vi "NI 5772 (AC) - Digitizer_(FPGA)AveragingTesting.vi"() -> ()   [LabVIEW 2020]
doc: "Example Description:\nThis example demonstrates how to enable Time Interleaved Sampling with the NI 5772 adapter module to achieve a sampling rate of 1.6GS/s. This example continuously acquires records of analog input data from the NI 5772 adapter module. It allows you to select an AI channel, trigger type, and record size. This VI must be compiled before it is run. \n\nRunning the VI:\nThis VI must be run from the NI 5772 - Getting Started (Host).vi. Refer to the host VI documentation for steps regarding running and configuring the FPGA VI. \n\nExecution Steps:\nRefer to the Block Diagram of this VI for execution comments."
uses:
  Controls/AI Trigger Type.ctl
  Controls/Aquire State.ctl
panel:
  in  "Trigger":bool=TRUE
  out "Trigger Count":u32
  out "Read Size (Host)":u16=512 caption="Samples Per Trigger" min=1 step=1
  in  "TrigIn Simulate":bool
  in  "vi/nGenTrig":bool
  in  "Arm Trigger":bool
  out "F to H FIFO Overflow?":bool caption="FIFO Overflow?"
  out "DataAlignmentFIFO":bool
  out "Aq to Trans FIFO Overflow?":bool caption="FIFO Overflow?"
  in  "Requested Samples Per Pixel":u16=512 caption="Samples Per Trigger" min=1 step=1
  in  "AvgCount_powerOf2":i16=1
  in  "Delay (us)":sgl
  in  "WaveSampleCount":sgl=256.0 format="%#_13g"
  in  "Wave Sampling Rate":sgl=200000000.0 format="%#_6p"
  in  "Trigger Level":i16
  in  "Trigger Type":T1
  out "AvgCount":u16=1
  out "Delay after Trig [cycles]":u16
  out "1/8th Samples Per Trigger":u16=512 caption="Samples Per Trigger" min=1 step=1
  out "WaitForWave\nCompletion [cycles]":u16
  in  "User Command Commit":bool
  in  "User Command":u8
  out "User Command Idle":bool
  out "User Command Status":u8
  in  "User Data 0":u16
  in  "User Data 1":u8
  out "PLL Locked":bool
  out "User Error":bool
  out "Configured?":bool
  # "Trigger Settings"
  # "FIFO Status"
  # "Analog Input"
  # "Clock Configuration"
  # "Resource Configuration"
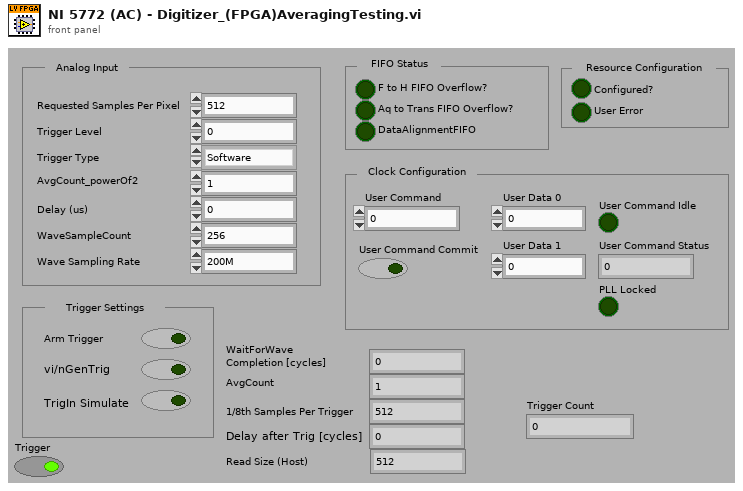
[diagram p1: front panel]
types:
  T1 = typedef "AI Trigger Type.ctl" = enum8{"Software", "Data Edge"}
  T2 = typedef "Aquire State.ctl" = enum8{"Idle", "Wait for Trigger", "AlignWave", "Hold Aquire", "Acquire", "WaitForWaveCompletion", "CheckAvg"}
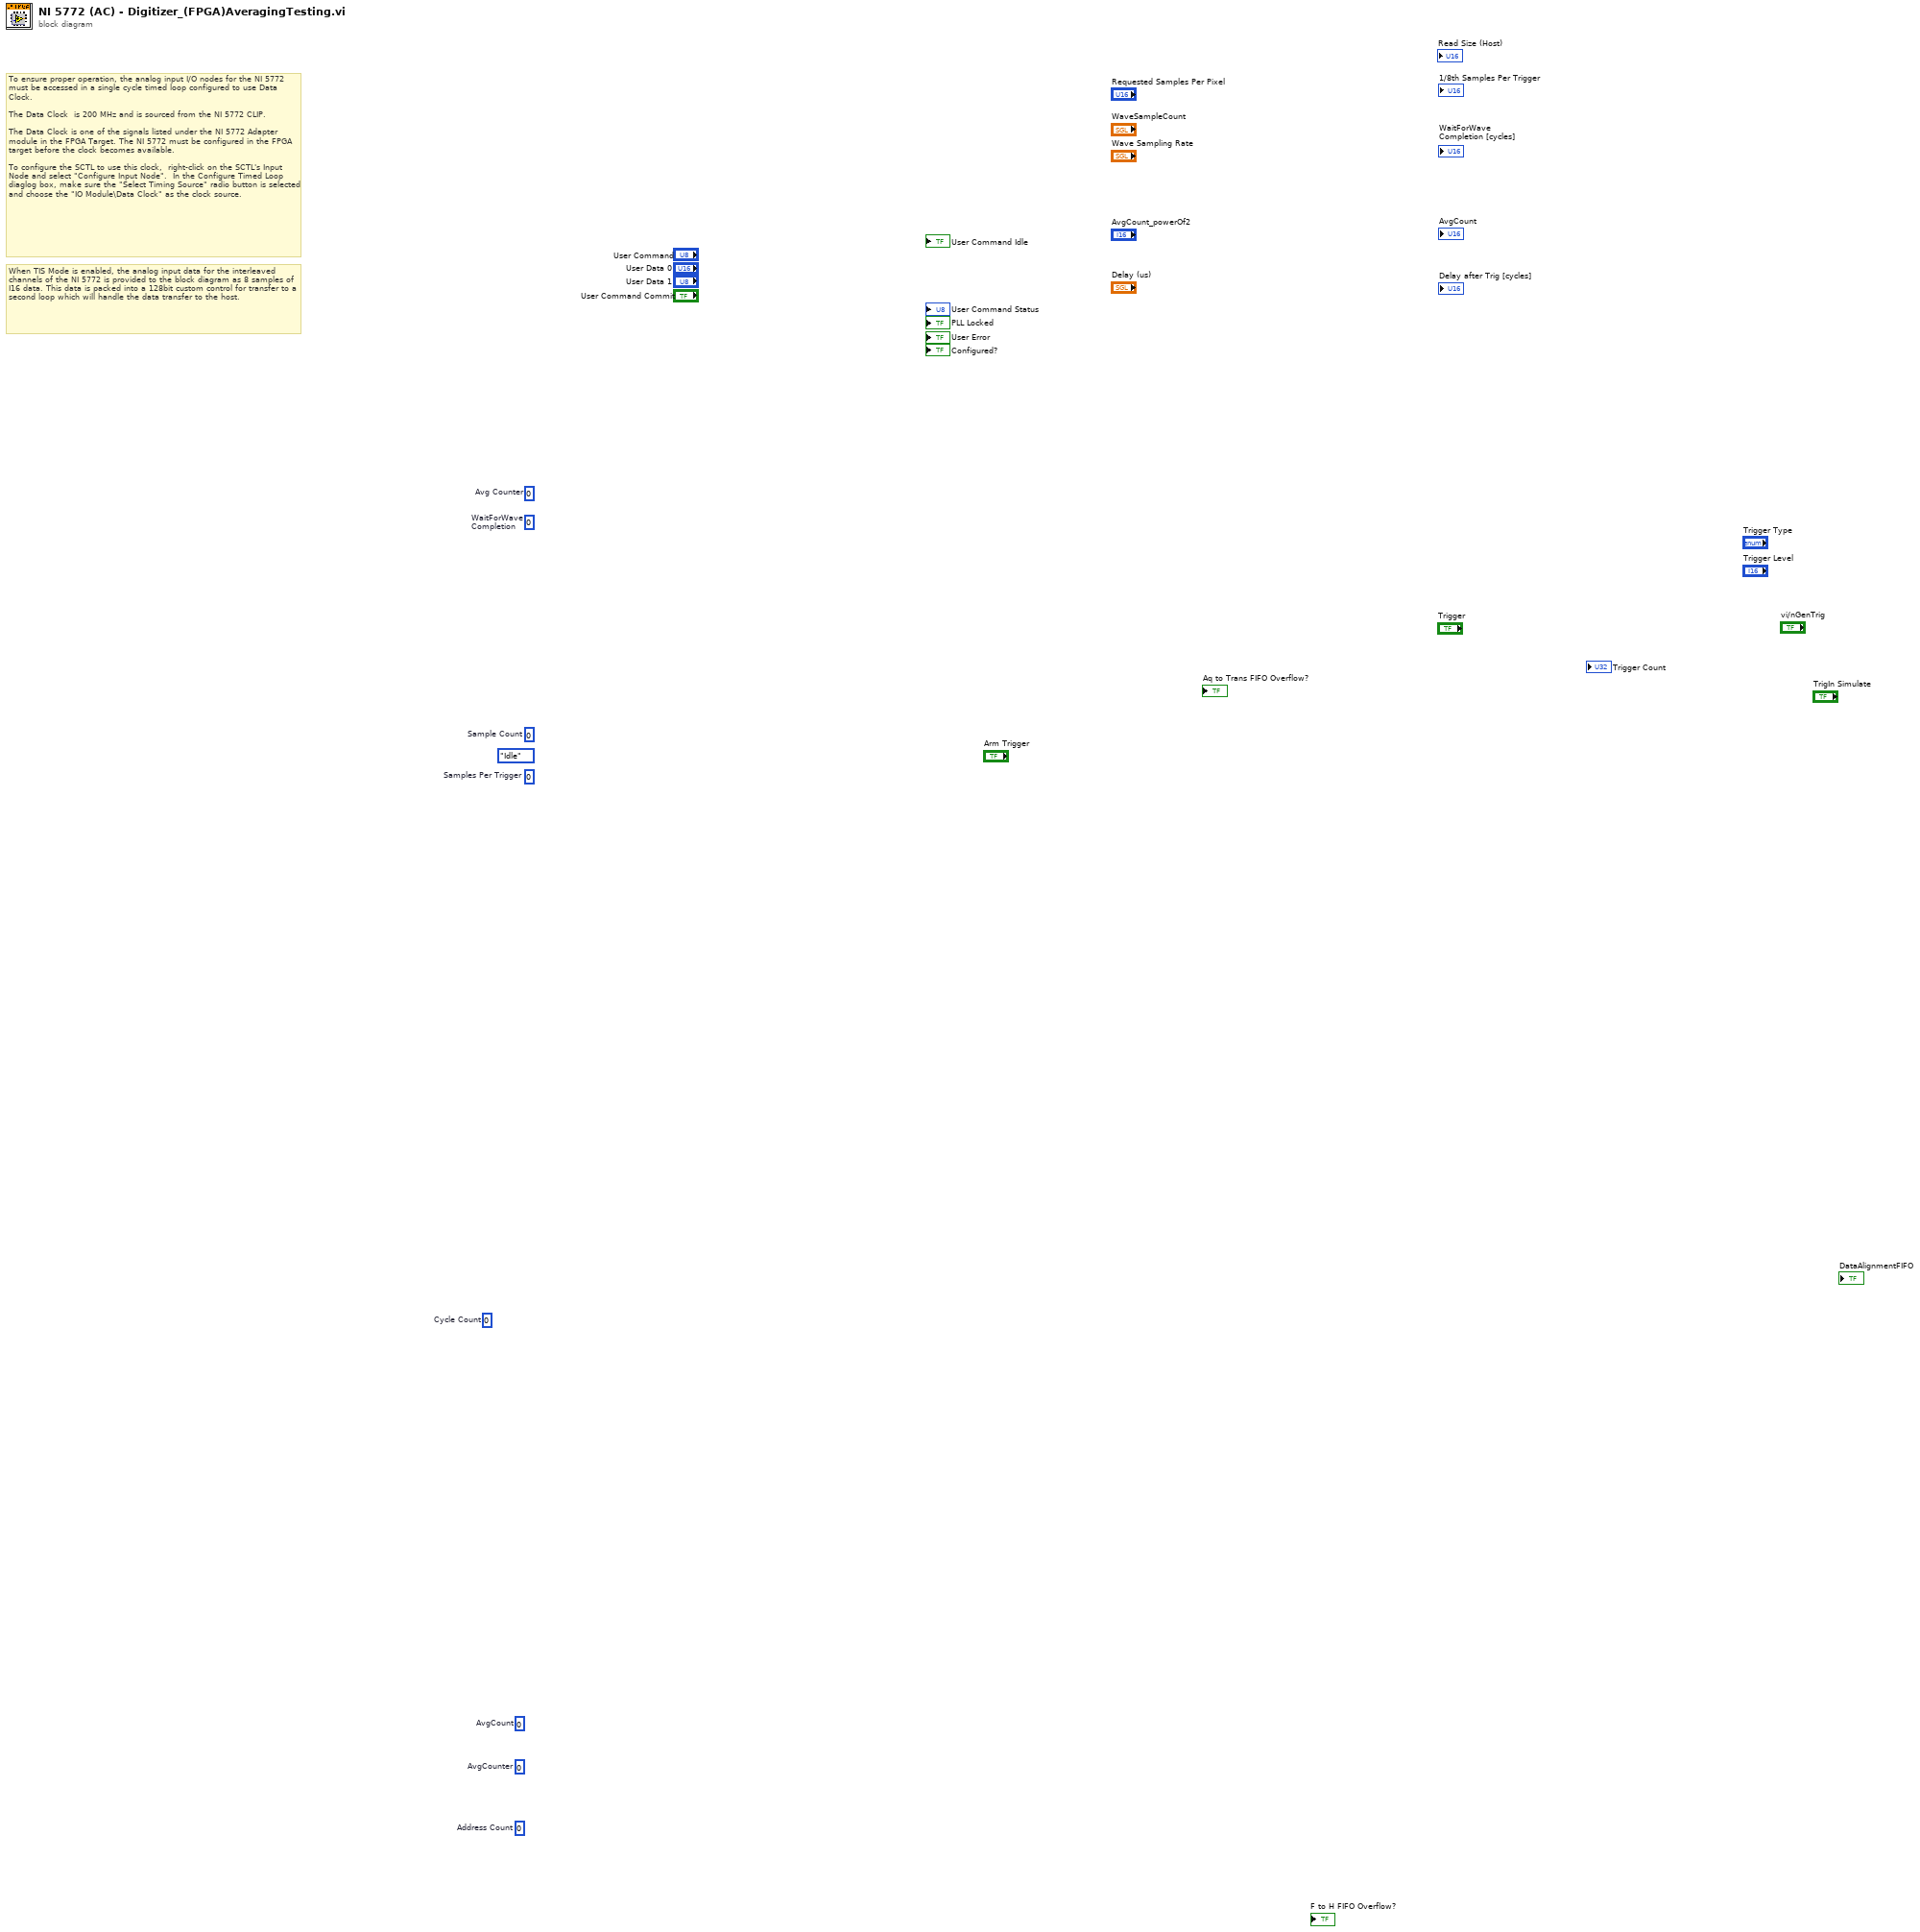
[diagram p0: block diagram]
diagram:
  (unwired) u16 0  # Cycle Count
  (unwired) u16 0  # AvgCounter
  (unwired) u32 0  # Address Count
  (unwired) u16 0  # AvgCount
  (unwired) u16 0  # WaitForWave Completion
  (unwired) u16 0  # Avg Counter
  (unwired) u16 0  # Samples Per Trigger
  (unwired) u16 0  # Sample Count
  (unwired) Aquire_State."Idle" ("Acquire State")
  # "When TIS Mode is enabled, the analog input data for the interleaved channels of the NI 5772 is provided to the block diagram as 8 samples of I16 data. This data is packed into a 128bit custom control for transfer to a second loop which will handle the data transfer to the host."
  # "To ensure proper operation, the analog input I/O nodes for the NI 5772 must be accessed in a single cycle timed loop configured to use Data Clock. \n\nThe Data Clock  is 200 MHz and is sourced from the NI 5772 CLIP.\n\nThe Data Clock is one of the signals listed under the NI 5772 Adapter module in the FPGA Target. The NI 5772 must be configured in the FPGA target before the clock becomes available. \n\nTo configure the SCTL to use this clock,  right-click on the SCTL's Input Node and select \"Configure Input Node\".  In the Configure Timed Loop diaglog box, make sure the \"Select Timing Source\" radio button is selected and choose the \"IO Module\\Data Clock\" as the clock source."
